vi "Unbundle.vi"(8 "error in":errorcluster, 11 "Instrument List Data in":refnum<class "Instrument List Data.lvclass">) -> (0 "error out":errorcluster, 2 "Instrument Info Array":T1[](array[typedef]), 3 "Instrument List Data out":refnum<class "Instrument List Data.lvclass">)   [LabVIEW 2020, in "Instrument Handler.lvlib" / "Instrument List Data.lvclass"]
doc: "Read the Instrument List Data."
uses:
  Instrument List Data.lvclass
  Controls/Ctl_InstrumentInfo.ctl
  Instrument List Data.lvclass/Instrument List Data.ctl
  Instrument Handler.lvlib
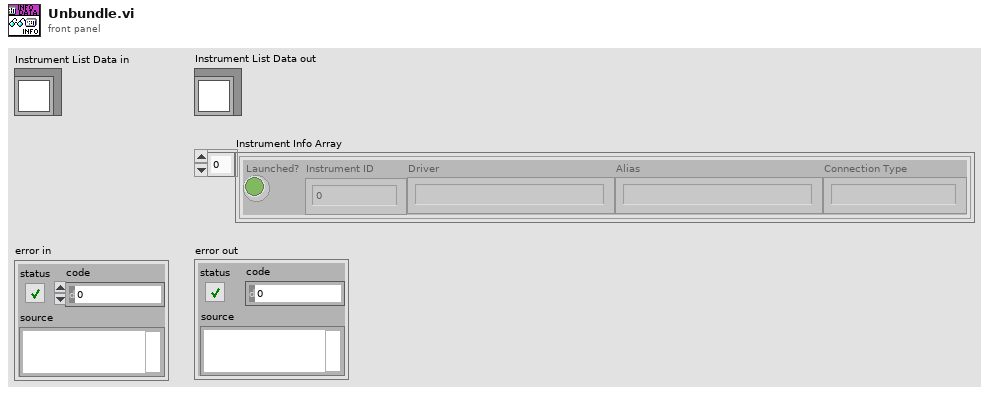
[diagram p1: front panel]
types:
  T1 = typedef "Instrument Handler.lvlib/Ctl_InstrumentInfo.ctl" = cluster{"Launched?":bool, "Instrument ID":u32, "Driver":string, "Alias":string, "Connection Type":string}
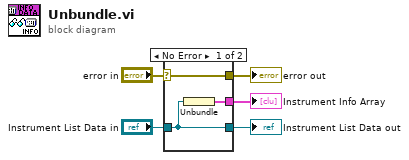
[diagram p0: block diagram]
diagram:
  n1 = case shown="No Error" "error in" {
    selector: "error in" -> [w7 w9]
    tunnel: [w6 w10] -> w5
    tunnel: "Instrument List Data in" -> [w6 w10]
    tunnel: [w8 _] -> w3
    tunnel: [w7 w9] -> w1
    frame No Error {
      n2 = Unbundle(w6) -> (w8:T1[])
    }
    frame Error {
    }
  }
  "Instrument List Data out" <- w5
  "Instrument Info Array" <- w3
  "error out" <- w1
